vi "UploadAcquisitions.vi"(6 "test slug":string, 7 "step id":i32, 8 "error in (no error)":errorcluster, 9 "acquisitions":T1[](array[typedef]) {"timestamp" format="%<%x %.3X>T"}, 10 "asset code":string, 11 "ByteQXAPIBase in":refnum<class "ByteQXAPIBase.lvclass">) -> (0 "error out":errorcluster, 3 "ByteQXAPIBase out":refnum<class "ByteQXAPIBase.lvclass">)   [LabVIEW 2019, in "ByteQXWebAPI.lvlib" / "ByteQXAPIBase.lvclass"]
doc: "Uploads data acquired from an asset\nIt can be a test-related data. In that case, it needs step id and test slug both taken from the specific test.\nOtherwise, it can be just logged data, leaving step id and test slug empty"
uses:
  ByteQXAPIBase.lvclass
  Acquisitions.ctl
  Private/module.ctl
  LimsTestStep/UploadAcquisitions_ReqData.ctl
  Acquisition_ReqData.ctl
  <vilib>/Bytelabs/ByteREST/ByteRESTClass/ByteRESTBase/HTTP/Status_Code.ctl
  ByteQXAPIBase.lvclass/ByteQXAPIBase.ctl
  <vilib>/Bytelabs/ByteREST/ByteRESTClass/ByteRESTBase/RESTBase.lvclass
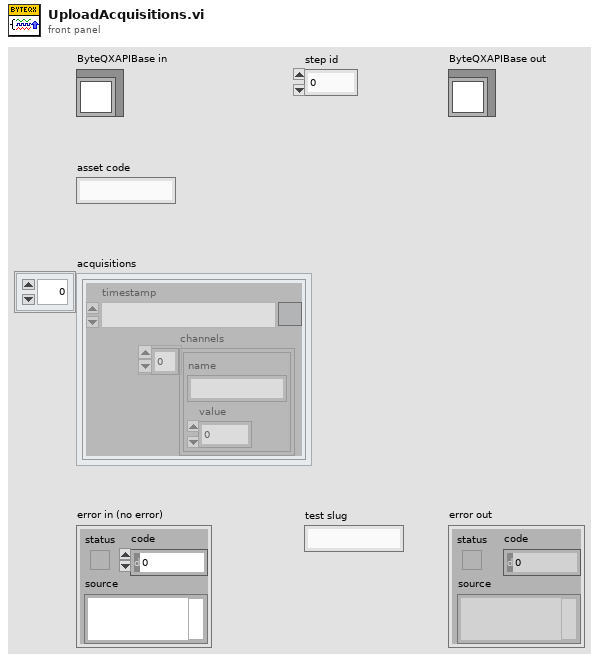
[diagram p1: front panel]
types:
  T1 = typedef "ByteQXWebAPI.lvlib/ByteQXAPIBase.lvclass/Acquisitions.ctl" = cluster{"timestamp":timestamp, "channels":cluster{"name":string, "value":dbl}[]}
  T2 = typedef "ByteQXWebAPI.lvlib/ByteQXAPIBase.lvclass/UploadAcquisitions_ReqData.ctl" = cluster{"tags":cluster{"step_id":i32, "test_slug":string, "asset_slug":string}, "acquisitions":T3[]}
  T3 = typedef "ByteQXWebAPI.lvlib/ByteQXAPIBase.lvclass/Acquisition_ReqData.ctl" = cluster{"timestamp":string, "fields":cluster{"name":string, "value":dbl}[]}
  T4 = typedef "ByteQXWebAPI.lvlib/ByteQXAPIBase.lvclass/module.ctl" = enum16{"gs", "tms", "data"}
  T5 = typedef "ByteREST.lvlib/RESTBase.lvclass/Status_Code.ctl" = u16
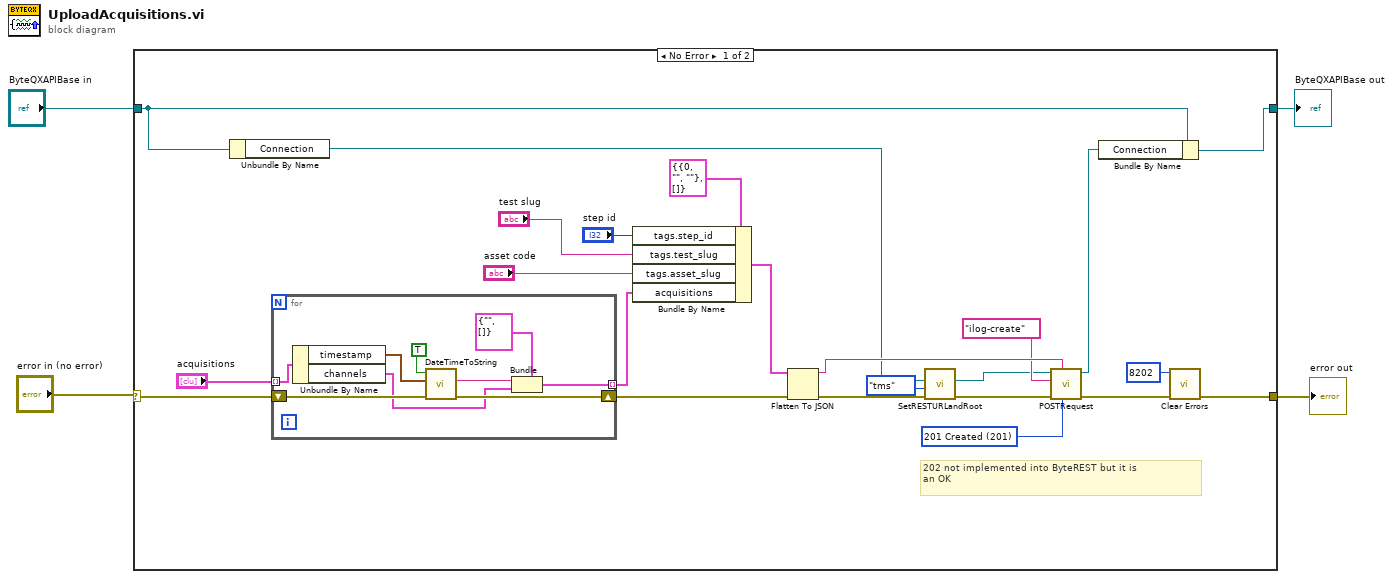
[diagram p0: block diagram]
diagram:
  n1 = case shown="No Error" "error in (no error)" {
    selector: "error in (no error)" -> [w11 w38]
    tunnel: [w6 w38] -> w3
    tunnel: [w26 w37] -> w1
    tunnel: "ByteQXAPIBase in" -> [w27 w37]
    frame No Error {
      w7 = T5 201 items=["200 OK"=200, "201 Created"=201, "400 Bad Request"=400, "401 Unauthorized"=401, "403 Forbidden"=403, "404 Not Found"=404, "405 Method Not Allowed"=405, "406 Not Acceptable"=406, "500 Internal Server Error"=500] ("expected response")
      # "202 not implemented into ByteREST but it is \nan OK"
      n2 = Unbundle By Name(w27) -> ("Connection"=w18:refnum<class "RESTBase.lvclass">)
      n3 = for {
        shift-right: [w34] -> w10
        shift-left: w11 -> [w35]
        tunnel: "acquisitions" -> [w33] mode=indexing
        tunnel: [w29] -> w8 mode=indexing
        n4 = Unbundle By Name(w33) -> ("timestamp"=w32:timestamp, "channels"=w30:cluster{"name":string, "value":dbl}[])
        n5 = call "DateTimeToString.vi"("error in"=w35, "current time"=w32, "include Time?"=TRUE) -> ("error out"=w34:errorcluster, "date string"=w31:string)  [unwired: 7 in]
        n6 = Bundle(cluster=T3 {"timestamp"="", "fields"=[]} ("Cluster"), "timestamp"=w31, "fields"=w30) -> (w29:T3)
      }
      n7 = Bundle By Name(cluster=T2 {"tags"={"step_id"=0, "test_slug"="", "asset_slug"=""}, "acquisitions"=[]} ("Acquisitions"), "tags.step_id"="step id", "tags.test_slug"="test slug", "tags.asset_slug"="asset code", "acquisitions"=w8) -> (w15:T2)
      n8 = Flatten To JSON(anything=w15, error in (no error)=w10) -> (JSON string=w25:string, 11:w20:errorcluster)  [unwired: 1 in]
      n9 = call "SetRESTURLandRoot.vi"("error in (no error)"=w20, "module"=module."tms", "ByteREST in"=w18) -> ("error out"=w19:errorcluster, "ByteREST out"=w17:refnum<class "RESTBase.lvclass">)  [unwired: 7 in]
      n10 = call-dynamic "POSTRequest.vi"("expected response"=w7, "Body in"=w25, "error in (no error)"=w19, "Request"="ilog-create", "ByteRESTBase in"=w17) -> ("error out"=w22:errorcluster, "ByteRESTBase out"=w24:refnum<class "RESTBase.lvclass">)  [unwired: 3 in, 2 out]
      n11 = Bundle By Name(cluster=w27, "Connection"=w24) -> (w26:refnum<class "ByteQXAPIBase.lvclass">)
      n12 = call <vilib>:"Clear Errors.vi"("error in (no error)"=w22, "specific error code to clear (0: all)"=8202) -> ("error out"=w6:errorcluster)  [unwired: 4 in, 1 out]
    }
    frame Error {
    }
  }
  "error out" <- w3
  "ByteQXAPIBase out" <- w1
